vi "setName.vi"(8 "error in (no error)":errorcluster, 10 "name":string, 11 "reference in":refnum<class "subject.lvclass">) -> (0 "error out":errorcluster, 3 "reference out":refnum<class "subject.lvclass">)   [LabVIEW 2015, in "subject.lvclass"]
uses:
  subject.lvclass
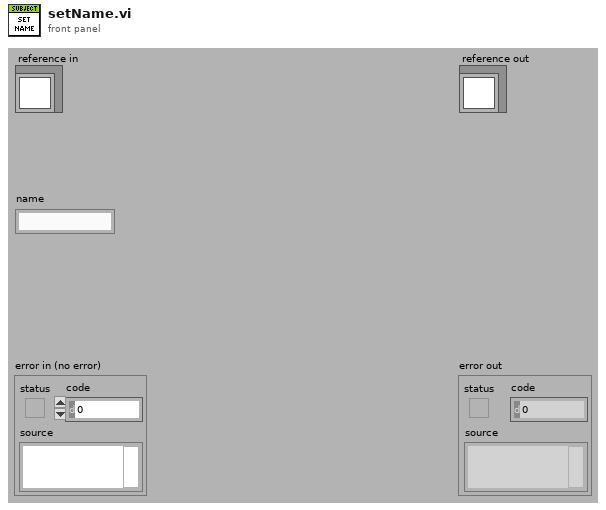
[diagram p1: front panel]
types:
  T1 = typedef "subject.lvclass/ObjectAttributesRef.ctl" = refnum<data-value>
  T2 = typedef "subject.lvclass/ObjectAttributes.ctl" = cluster{"MyAttribute":dbl, "data":cluster{"Ve_warm":dbl[], "time_warm":dbl[], "name":string, "phase":dbl[], "VCO2":dbl[], "VO2":dbl[], "PetCO2":dbl[], "RQ":dbl[], "HR":dbl[], "Ve_warm_inter":dbl[], "time_warm_inter":dbl[], "Ve_exer":dbl[], "time_exer":dbl[], "Ve_exer_inter":dbl[], "time_exer_inter":dbl[], "Ve":dbl[], "time":dbl[], "Ve_exer_inter_filtered":dbl[], "Ve_warm_inter_filtered":dbl[]}, "results_5l":cluster{"EOV":bool, "osci_amplitude":dbl[], "osci_width":dbl[], "peak_location":dbl[], "threshold":dbl, "width":i32}, "results_15percent":cluster{"EOV":bool, "osci_amplitude":dbl[], "osci_width":dbl[], "peak_location":dbl[], "threshold":dbl, "width":i32}, "supportData":cluster{"peaksAmplitude":dbl[], "iPeaksLocation":dbl[], "valesAmplitude":dbl[], "iValesLocation":dbl[], "threshold":dbl, "meanAmpl_warm":i32, "#_peaks":i32, "width":i32}, "results_user_selection":cluster{"EOV":bool, "osci_amplitude":dbl[], "osci_width":dbl[], "peak_location":dbl[], "threshold":dbl, "width":i32}, "results_warm_up":cluster{"EOV":bool, "osci_amplitude":dbl[], "osci_width":dbl[], "peak_location":dbl[], "threshold":dbl, "width":i32}}
  T3 = typedef "subject.lvclass/ClassAttributesRef.ctl" = refnum<data-value>
  T4 = typedef "subject.lvclass/ClassAttributes.ctl" = cluster{"Dummy":bool, "subject_refs":refnum<class "subject.lvclass">[]}
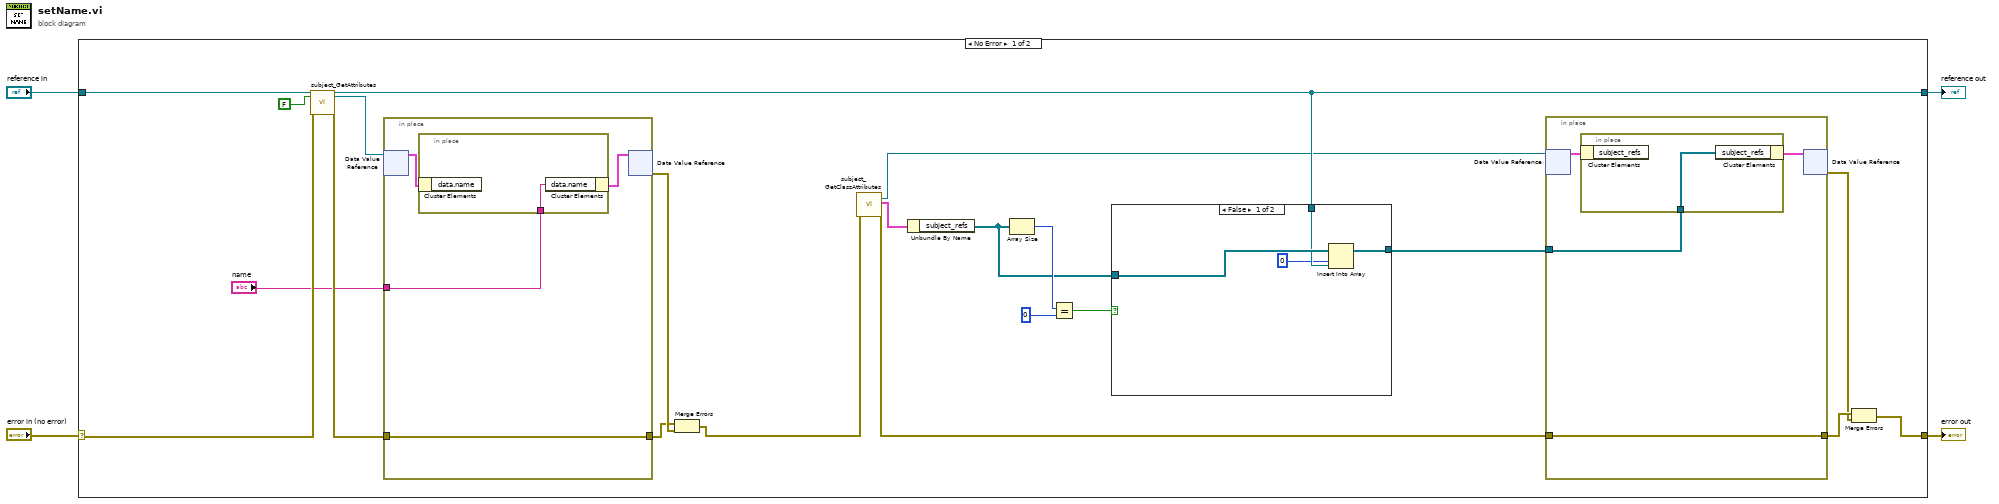
[diagram p0: block diagram]
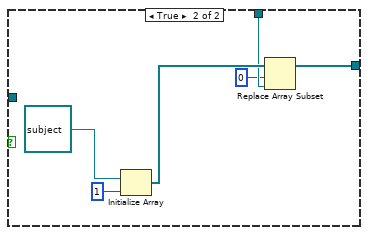
[diagram p2: hidden frame]
diagram:
  n1 = case shown="No Error" "error in (no error)" {
    selector: "error in (no error)" -> [w21 w47]
    tunnel: [w6 w47] -> w3
    tunnel: [w15 w46] -> w1
    tunnel: "reference in" -> [w23 w46]
    frame No Error {
      n2 = call "subject_GetAttributes.vi"("reference in"=w23, "return data? (T)"=FALSE, "error in (no error)"=w21) -> ("reference out"=w15:refnum<class "subject.lvclass">, "attributes ref"=w19:T1, "error out"=w20:errorcluster)  [unwired: 13 in, 1 out]
      n3 = in-place {
        in-place-border: w20 -> [w42]
        in-place-border: [w42] -> w24
        in-place-border: "name" -> [w41]
        n4 = in-place-dvr #1(w19) -> (w43:T2)  [unwired: 1 out]
        n5 = in-place {
          in-place-border: w41 -> [w45]
          n6 = in-place-cluster #2(w43) -> ()  [unwired: 1 out]
          n7 = in-place-cluster #2("data.name"=w45) -> (w44:T2)
        }
        n8 = in-place-dvr #1(w44) -> (w25:errorcluster)  [unwired: 1 out]
      }
      n9 = Merge Errors(w24, w25) -> (w10:errorcluster)
      n10 = call "subject_GetClassAttributes.vi"("error in (no error)"=w10) -> ("class attributes ref"=w12:T3, "class attributes"=w18:T4, "error out"=w13:errorcluster)  [unwired: 15 in, 1 out]
      n11 = Unbundle By Name(w18) -> ("subject_refs"=w14:refnum<class "subject.lvclass">[])
      n12 = Array Size(array=w14) -> (size(s)=w17:i32)
      n13 = Equal?(x=w17, y=0) -> (x = y?=w16:bool)
      n14 = case shown="False" w16 {
        tunnel: w15 -> [w32 w37]
        tunnel: w14 -> [w34 _]
        tunnel: [w33 w39] -> w11
        frame False {
          n15 = Insert Into Array(array=w34, index=0, new element=w32) -> (w33:refnum<class "subject.lvclass">[])
        }
        frame True {
          n16 = Initialize Array(refnum<class "subject.lvclass"> refnum ("subject.lvclass"), 1 ("dimension size")) -> (w40:refnum<class "subject.lvclass">[])
          n17 = Replace Array Subset(array=w40, new element=w37, index=0) -> (w39:refnum<class "subject.lvclass">[])
        }
      }
      n18 = in-place {
        in-place-border: w13 -> [w27]
        in-place-border: [w27] -> w7
        in-place-border: w11 -> [w26]
        n19 = in-place-dvr #3(w12) -> (w28:T4)  [unwired: 1 out]
        n20 = in-place {
          in-place-border: w26 -> [w30]
          n21 = in-place-cluster #4(w28) -> ()  [unwired: 1 out]
          n22 = in-place-cluster #4("subject_refs"=w30) -> (w29:T4)
        }
        n23 = in-place-dvr #3(w29) -> (w5:errorcluster)  [unwired: 1 out]
      }
      n24 = Merge Errors(w7, w5) -> (w6:errorcluster)
    }
    frame Error {
    }
  }
  "error out" <- w3
  "reference out" <- w1
